vi "move V2.0.vi"(8 "error in (no error)":errorcluster, 9 "RPM":dbl, 10 "Y":dbl, 11 "X":dbl) -> (0 "error out":errorcluster)   [LabVIEW 2019]
uses:
  <vilib>/Platform/TimedLoop/XDataNode/timing_clust.ctl
  <vilib>/Platform/TimedLoop/XDataNode/nitl_modes.ctl
  <vilib>/Platform/TimedLoop/XDataNode/wakeup.ctl
  <vilib>/platform/TimedLoop/XDataNode/XDataNode.xnode
  <vilib>/Platform/TimedLoop/XDataNode/XDNodeRunTimeDep.lvlib
panel:
  out "AC estimate (Vrms)":dbl format="%0.2f"
  out "out array":dbl[](array[numeric])
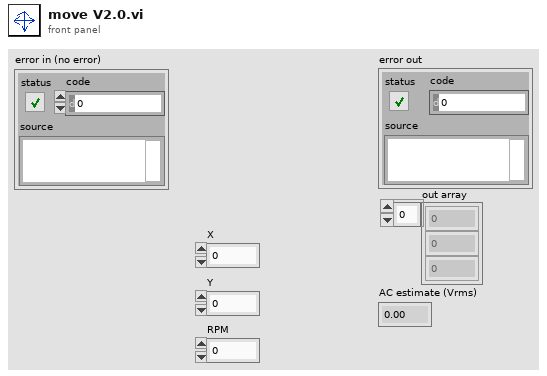
[diagram p1: front panel]
types:
  T1 = typedef "BNO055 gyro 3axis.ctl" = cluster{"yaw":dbl, "pitch":dbl, "roll":dbl}
  T2 = typedef "XDNodeRunTimeDep.lvlib/timing_clust.ctl" = cluster{"Expected End [f-1]":u64, "Actual End [f-1]":u64, "Finished Late? [f-1]":bool, "Expected End [i-1]":u64, "Actual End [i-1]":u64, "Finished Late? [i-1]":bool, "Expected Start [i]":u64, "Actual Start [i]":u64, "Expected Start [f]":u64, "Actual Start [f]":u64, "Source Name":string, "Structure Name":string, "Period":i64, "Deadline":i64, "Offset":i64, "Start":i64, "Priority":i32, "Timeout":i32, "Mode":T3, "Wakeup Reason":T4, "Error":errorcluster, "Source Type":string, "Secondary Source Type":string, "Global End Time":u64, "Global Start Time":u64, "Frame Duration":u64, "Iteration Duration":u64, "Assigned CPU":i32, "I/O Scan Engine Mode":u32}
  T3 = typedef "XDNodeRunTimeDep.lvlib/nitl_modes.ctl" = enum32{"No Change", "Process missed periods, maintain original phase", "Discard missed periods, maintain original phase", "Process missed periods, ignore original phase", "Discard missed periods, ignore original phase"}
  T4 = typedef "XDNodeRunTimeDep.lvlib/wakeup.ctl" = enum32{"Normal", "Aborted", "Asynchronous wakeup", "Timing source error", "Timed loop error", "Timeout"}
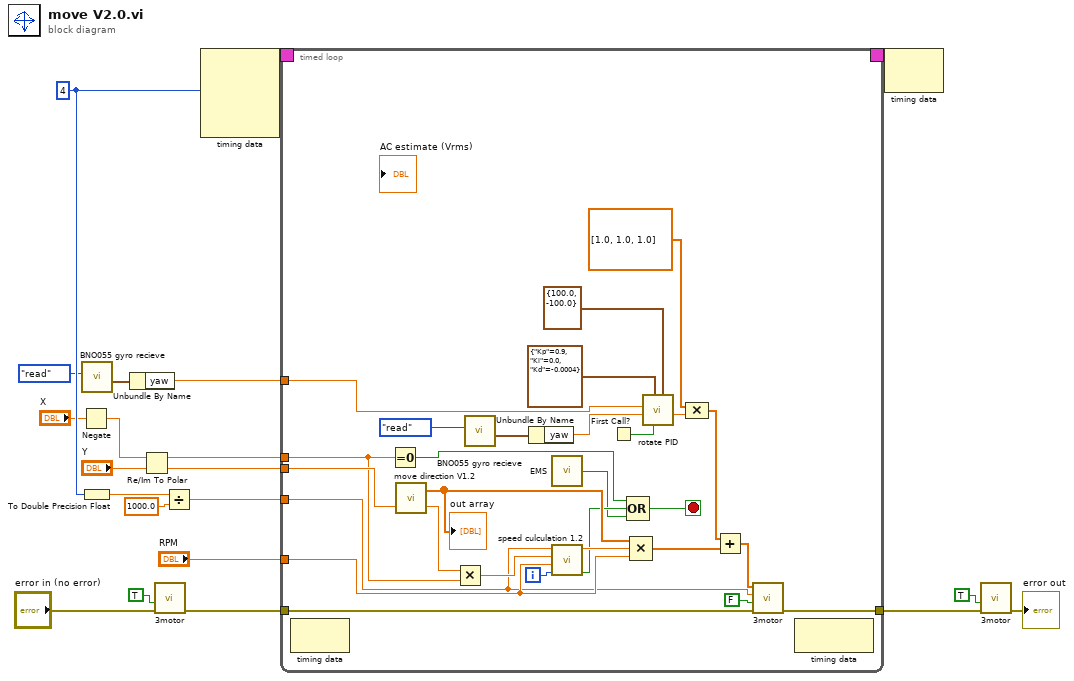
[diagram p0: block diagram]
diagram:
  w19 = i64 4 ("Period")
  n1 = Negate(x="X") -> (-x=w6:dbl)
  n2 = call "BNO055 gyro recieve.vi"("Enum"=enum16{"read", "write"}."read") -> ("read"=w2:T1)  [unwired: 10 in]
  n3 = To Double Precision Float(number=w19) -> (double precision float=w18:dbl)
  n4 = Unbundle By Name(w2) -> ("yaw"=w1:dbl)
  n5 = Re/Im To Polar(2:"Y", 3:w6) -> (0:w14:dbl, 1:w13:dbl)
  n6 = call "3motor.vi"("error in (no error)"="error in (no error)", "Reset"=TRUE) -> ("error out"=w11:errorcluster)  [unwired: 8 in, 1 out]
  n7 = Divide(x=w18, y=1000.0) -> (x/y=w16:dbl)
  n8 = node-c288(w19) -> (w21:T2)  [unwired: 3 in]
  n9 = timed-loop {
    timing: w21 -> [_]
    timing-out: [_] -> w20
    tunnel: w16 -> [w31]
    tunnel: w14 -> [w48]
    tunnel: w13 -> [w34]
    tunnel: "RPM" -> [w39]
    tunnel: w11 -> [w33]
    tunnel: [w46] -> w5
    tunnel: w1 -> [w24]
    i -> [w49]
    stop <- w36 stop-if-true
    n10 = node-c288() -> ()  [unwired: 1 in, 1 out]
    n11 = Equal To 0?(x=w34) -> (x = 0?=w35:bool)
    n12 = call "move direction V1.2.vi"("theta"=w48) -> ("max value"=w40:dbl, "out array"=w47:dbl[])  [unwired: 1 in]
    "out array" <- w47
    n13 = Multiply(x=w40, y=w34) -> (x*y=w41:dbl)
    n14 = call "BNO055 gyro recieve.vi"("Enum"=enum16{"read", "write"}."read") -> ("read"=w27:T1)  [unwired: 10 in]
    n15 = Unbundle By Name(w27) -> ("yaw"=w25:dbl)
    n16 = call "EMS.vi"() -> ("A/DIO4 (Pin 19)"=w32:bool)
    n17 = call "speed culculation 1.2.vi"("i"=w49, "Speed(RPM)"=w39, "distance"=w41, "dt(s)"=w31) -> ("complet?"=w37:bool, "Speed"=w43:dbl)  [unwired: 4 in, 2 out]
    n18 = First Call?() -> (First Call?: T/F=w28:bool)
    n19 = Compound Arithmetic op=OR(w35, w37, w32) -> (w36:bool)
    n20 = Compound Arithmetic op=MULTIPLY(w47, w43, w39) -> (w45:dbl[])
    n21 = call "rotate PID.vi"("output range"=cluster{"output high":dbl, "output low":dbl} {"output high"=100.0, "output low"=-100.0}, "s"=w28, "PID"=cluster{"Kp":dbl, "Ki":dbl, "Kd":dbl} {"Kp"=0.9, "Ki"=0.0, "Kd"=-0.0004}, "Processer"=w25, "setpoint"=w24) -> ("out"=w23:dbl)  [unwired: 5 in, 1 out]
    n22 = Compound Arithmetic op=MULTIPLY(dbl[] [1.0, 1.0, 1.0], w23) -> (w44:dbl[])
    n23 = Add(x=w44, y=w45) -> (x+y=w42:dbl[])
    n24 = call "3motor.vi"("error in (no error)"=w33, "Reset"=FALSE, "dt(s)"=w31, "Motor speed"=w42) -> ("error out"=w46:errorcluster)  [unwired: 6 in, 1 out]
    n25 = node-c288() -> ()  [unwired: 1 in, 1 out]
  }
  n26 = node-c288(w20) -> ()  [unwired: 1 out]
  n27 = call "3motor.vi"("error in (no error)"=w5, "Reset"=TRUE) -> ("error out"=→"error out":errorcluster)  [unwired: 8 in, 1 out]
